vi "Recieve New Subscription.vi"(8 "error in (no error)":errorcluster, 9 "Topic":string, 10 "Name":string, 11 "Simple Chat in":refnum<class "Simple Chat.lvclass">) -> (0 "error out":errorcluster, 3 "Simple Chat out":refnum<class "Simple Chat.lvclass">)   [LabVIEW 2020, in "Simple Chat.lvlib" / "Simple Chat.lvclass"]
uses:
  Simple Chat.lvclass
  Simple Chat.lvclass/Simple Chat.ctl
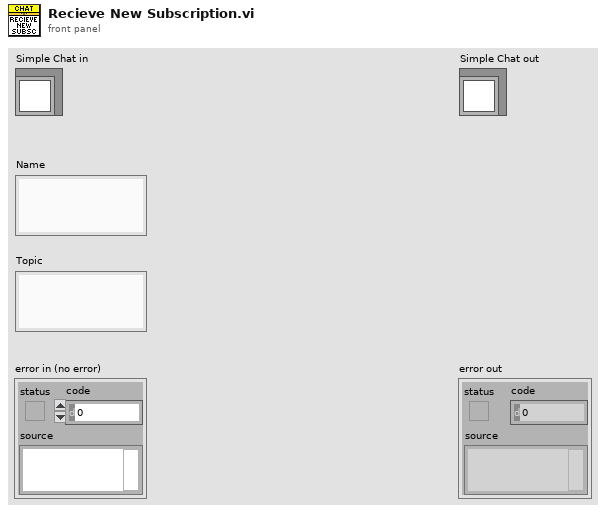
[diagram p1: front panel]
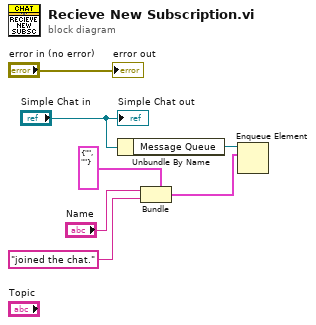
[diagram p0: block diagram]
diagram:
  n1 = Unbundle By Name("Simple Chat in") -> ("Message Queue"=w6:refnum<queue>)
  n2 = Bundle(cluster=cluster{"Sender":string, "Message":string} {"Sender"="", "Message"=""} ("element"), "Sender"="Name", "Message"="joined the chat.") -> (w4:cluster{"Sender":string, "Message":string})
  n3 = Enqueue Element(queue=w6, element=w4) -> ()  [unwired: 2 in, 3 out]
  "error out" <- "error in (no error)"
  "Simple Chat out" <- "Simple Chat in"
